vi "试剂余量展示.vi"(11 "波形图 2":refnum<vi>) -> (3 "波形图":sgl[][](graph))   [LabVIEW 2016, in "斯坦道氨氮.lvlib"]
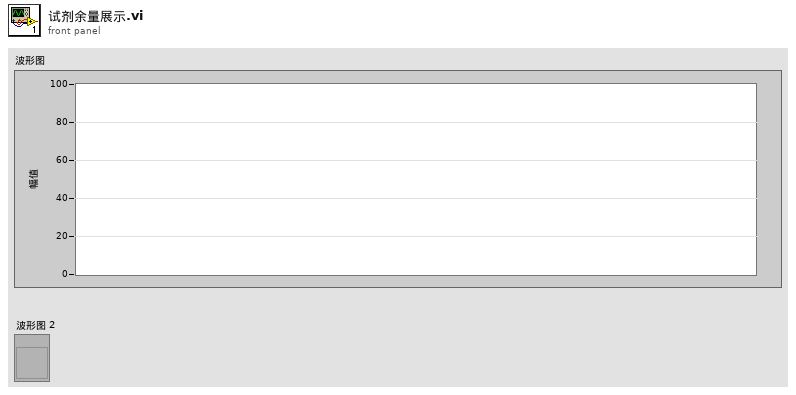
[diagram p1: front panel]
types:
  T1 = cluster{"V1":sgl, "V2":sgl, "V3":sgl, "V4":sgl, "V5":sgl, "V6":sgl, "V7":sgl, "V8":sgl, "V9":sgl, "V10":sgl, "V11":sgl, "V12":sgl, "V9-1":sgl, "V9-2":sgl}
  T2 = cluster{"V":string, "V 2":string, "V 3":string, "V 4":string, "V 5":string, "V 6":string, "V 7":string, "V 8":string, "V 9":string, "V 10":string, "V 11":string, "V 12":string, "V9-1":string, "V9-2":string}
  T3 = cluster{"Name":string, "Color":u32, "Style":u8, "Point Style":u8, "Name Visible":bool, "Allow Drag":bool, "Annotation Mode":u32, "Plot":i32, "Index":i32, "Position":cluster{"X":dbl, "Y":dbl}, "X Scale":u32, "Y Scale":u32, "Show Arrow":bool, "Lock Name":bool, "Plot Area":i32, "Label Offset":cluster{"X":dbl, "Y":dbl}}
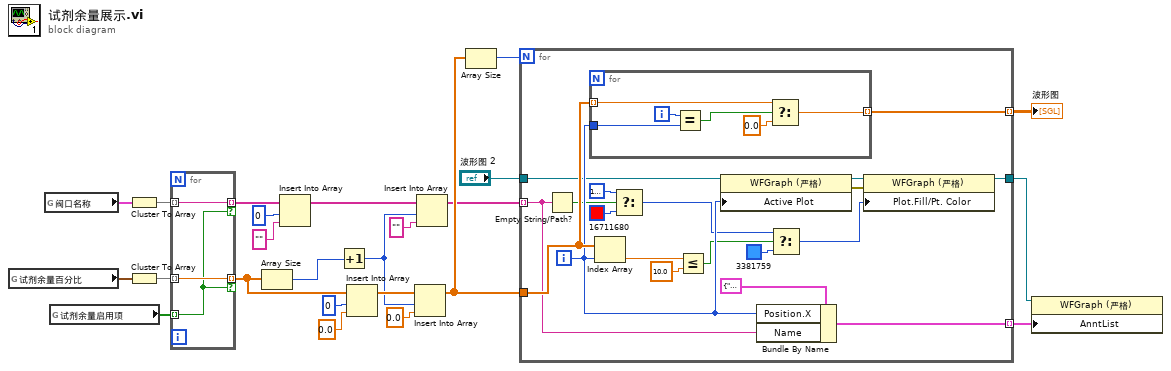
[diagram p0: block diagram]
diagram:
  n1 = global read "VAR总磷总氮全局变量.vi" "试剂余量百分比"() -> (w24:T1)
  n2 = global read "总磷总氮断电保存全局变量.vi" "阀口名称"() -> (w13:T2)
  n3 = global read "VAR总磷总氮全局变量.vi" "试剂余量启用项"() -> (w22:bool[])
  n4 = Cluster To Array(cluster=w13) -> (array=w12:string[])
  n5 = Cluster To Array(cluster=w24) -> (array=w23:sgl[])
  n6 = for {
    tunnel: w23 -> [w27] mode=indexing
    tunnel: w22 -> [w25] mode=indexing
    tunnel: [w27] -> w21 mode=indexing if=w25
    tunnel: w12 -> [w26] mode=indexing
    tunnel: [w26] -> w10 mode=indexing if=w25
  }
  n7 = Array Size(array=w21) -> (size(s)=w7:i32)
  n8 = Insert Into Array(array=w10, index=0 ("索引"), new element="" ("新元素/子数组")) -> (w8:string[])
  n9 = Increment(x=w7) -> (x+1=w3:i32)
  n10 = Insert Into Array(array=w21, index=0 ("索引"), new element=sgl 0.0 ("新元素/子数组")) -> (w19:sgl[])
  n11 = Insert Into Array(array=w19, index=w3, new element=sgl 0.0 ("新元素/子数组")) -> (w15:sgl[])
  n12 = Insert Into Array(array=w8, index=w3, new element="" ("新元素/子数组")) -> (w4:string[])
  n13 = Array Size(array=w15) -> (size(s)=w16:i32)
  n14 = for {
    N: w16 -> [_]
    tunnel: w15 -> [w40]
    tunnel: [w46] -> w14 mode=indexing
    tunnel: [w44] -> w11 mode=indexing
    tunnel: w4 -> [w35] mode=indexing
    tunnel: "波形图 2" -> [w30]
    tunnel: [w28] -> w1
    i -> [w39]
    n15 = Empty String/Path?(string/path=w35) -> (empty?=w34:bool)
    n16 = for {
      tunnel: w40 -> [w49] mode=indexing
      tunnel: [w48] -> w46 mode=indexing
      tunnel: w39 -> [w52]
      i -> [w51]
      n17 = Equal?(x=w51, y=w52) -> (x = y?=w50:bool)
      n18 = Select(t=w49, s=w50, f=sgl 0.0) -> (s? t:f=w48:sgl)
    }
    n19 = Index Array(array=w40, index=w39) -> (element=w38:sgl)
    n20 = Select(t=u32 16777216, s=w34, f=u32 16711680) -> (s? t:f=w31:u32)
    n21 = Less Or Equal?(x=w38, y=sgl 10.0) -> (x <= y?=w36:bool)
    n22 = property on="属性节点" class="WFGraph (严格)"(reference=w30, "Active Plot"=w39) -> (reference out=w29:refnum<vi>, error out=w43:errorcluster)  [unwired: 1 in]
    n23 = Bundle By Name(cluster=T3 {"Name"="", "Color"=0, "Style"=0, "Point Style"=0, "Name Visible"=TRUE, "Allow Drag"=FALSE, "Annotation Mode"=0, "Plot"=0, "Index"=0, "Position"={"X"=0.0, "Y"=10.0}, "X Scale"=0, "Y Scale"=0, "Show Arrow"=FALSE, "Lock Name"=FALSE, "Plot Area"=0, "Label Offset"={"X"=0.0, "Y"=0.0}}, "Position.X"=w39, "Name"=w35) -> (w44:T3)
    n24 = Select(t=w31, s=w36, f=u32 3381759) -> (s? t:f=w42:u32)
    n25 = property on="属性节点" class="WFGraph (严格)"(reference=w29, error in=w43, "Plot.Fill/Pt. Color"=w42) -> (reference out=w28:refnum<vi>)  [unwired: 1 out]
  }
  "波形图" <- w14
  n26 = property on="属性节点" class="WFGraph (严格)"(reference=w1, "AnntList"=w11) -> ()  [unwired: 1 in, 2 out]
